vi "Absolute Encoder Close.vi"(8 "Error":errorcluster, 11 "Cluster":T1) -> ()   [LabVIEW 2023]
uses:
  Cluster_Absolute Encoder Ref.ctl
  <vilib>/Rock Robotics/SystemInterfaces/DutyCycle/FPGA_DutyCycleDevRef.ctl
  <vilib>/Rock Robotics/SystemInterfaces/DutyCycle/FPGA_DutyCycleIndex.ctl
  <vilib>/Rock Robotics/WPI/Counter/WPI_CounterDevRef.ctl
  <vilib>/Rock Robotics/SystemInterfaces/Counter/FPGA_CounterCtrSystemIndex.ctl
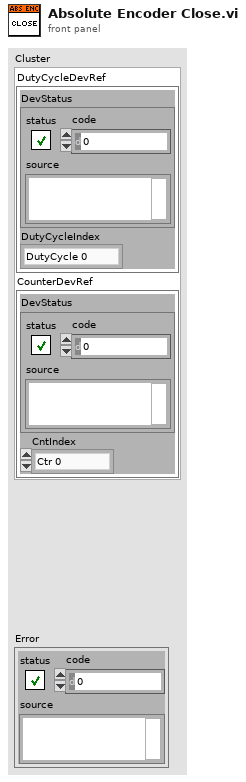
[diagram p1: front panel]
types:
  T1 = typedef "Cluster_Absolute Encoder Ref.ctl" = cluster{"DutyCycleDevRef":T2, "CounterDevRef":T4}
  T2 = typedef "FPGA_DutyCycleDevRef.ctl" = cluster{"DevStatus":errorcluster, "DutyCycleIndex":T3}
  T3 = typedef "FPGA_DutyCycleIndex.ctl" = enum8{"DutyCycle 0", "DutyCycle 1", "DutyCycle 2", "DutyCycle 3", "DutyCycle 4", "DutyCycle 5", "DutyCycle 6", "DutyCycle 7", "Invalid"}
  T4 = typedef "WPI_CounterDevRef.ctl" = cluster{"DevStatus":errorcluster, "CntIndex":T5}
  T5 = typedef "FPGA_CounterCtrSystemIndex.ctl" = enum8{"Ctr 0", "Ctr 1", "Ctr 2", "Ctr 3", "Ctr 4", "Ctr 5", "Ctr 6", "Ctr 7", "Invalid"}
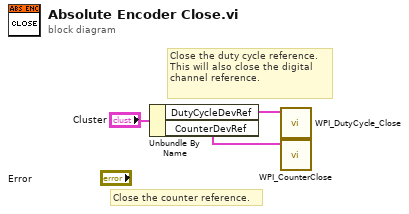
[diagram p0: block diagram]
diagram:
  # "Close the counter reference."
  # "Close the duty cycle reference.\nThis will also close the digital \nchannel reference."
  n1 = Unbundle By Name("Cluster") -> ("DutyCycleDevRef"=w2:T2, "CounterDevRef"=w3:T4)
  n2 = call <vilib>:"WPI_DutyCycle_Close.vi"("DutyCycleDevRef"=w2) -> ()  [unwired: 10 in, 1 out]
  n3 = call <vilib>:"WPI_CounterClose.vi"("CounterDevRef"=w3) -> ()  [unwired: 10 in, 1 out]
